vi "hadamard.vi"(1 "N":u16) -> (0 "Intensity Graph":dbl[][](graph))   [LabVIEW 2023]
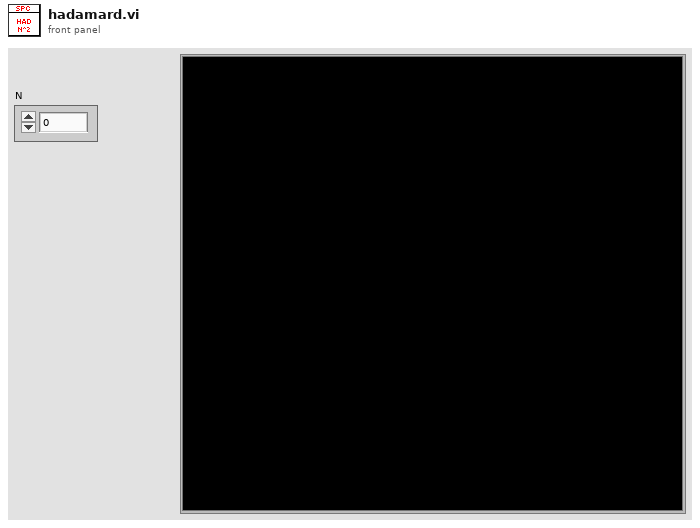
[diagram p1: front panel]
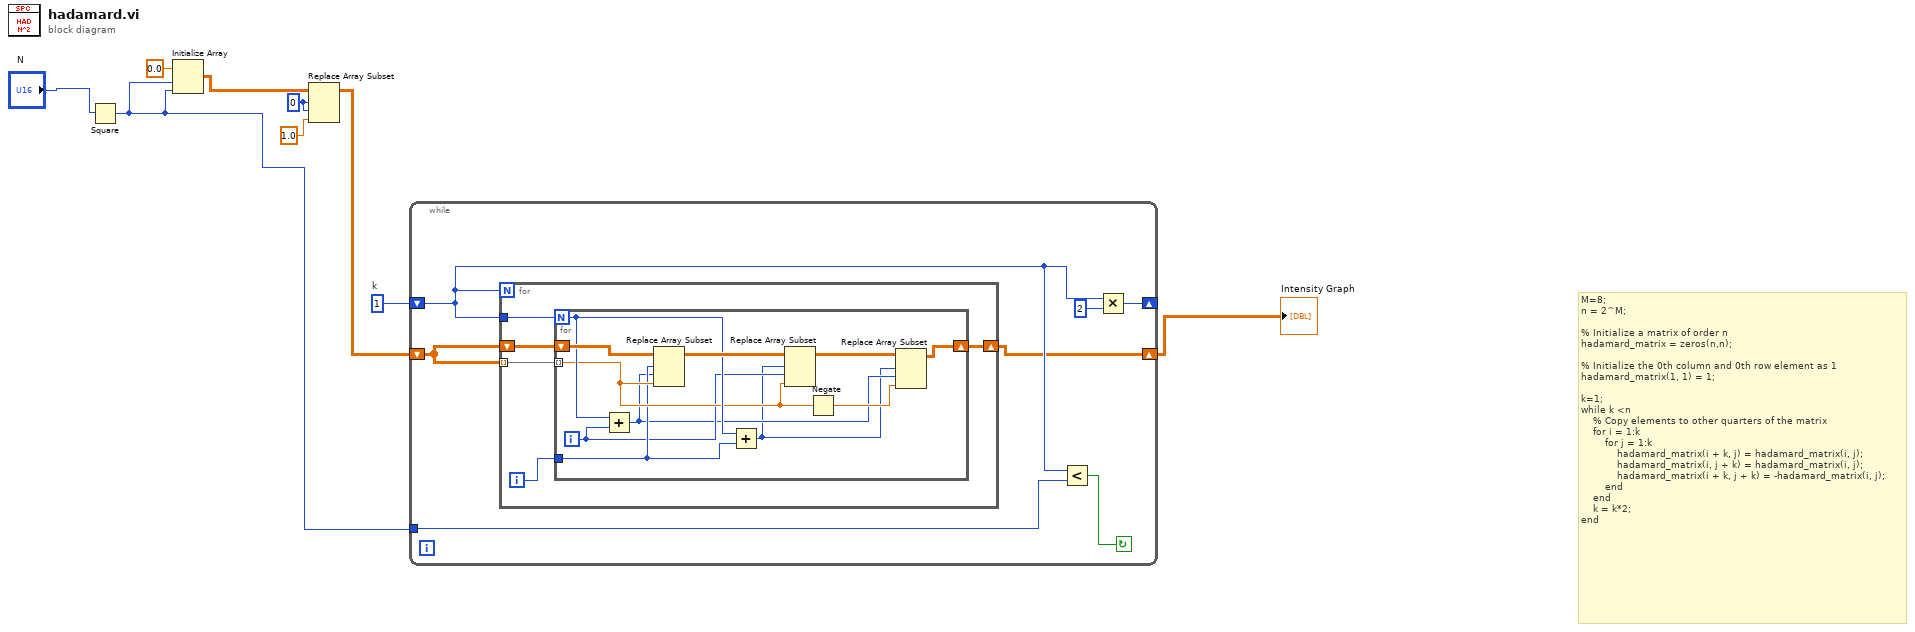
[diagram p0: block diagram]
diagram:
  w4 = 1  # k
  w6 = 0 ("index (row)")
  # "M=8;\nn = 2^M;\n\n% Initialize a matrix of order n\nhadamard_matrix = zeros(n,n);\n\n% Initialize the 0th column and 0th row element as 1\nhadamard_matrix(1, 1) = 1;\n\nk=1;\nwhile k <n\n    % Copy elements to other quarters of the matrix\n    for i = 1:k\n        for j = 1:k\n            hadamard_matrix(i + k, j) = hadamard_matrix(i, j);\n            hadamard_matrix(i, j + k) = hadamard_matrix(i, j);\n            hadamard_matrix(i + k, j + k) = -hadamard_matrix(i, j);\n        end\n    end\n    k = k*2;\nend"
  n1 = Square(x="N") -> (x^2=w2:u16)
  n2 = Initialize Array(0.0 ("element"), w2, w2) -> (w7:dbl[][])
  n3 = Replace Array Subset(array=w7, new element=1.0 ("new element/subarray"), index (row)=w6, index (col)=w6) -> (w3:dbl[][])
  n4 = while {
    shift-right: [w10] -> w1
    shift-left: w3 -> [w16]
    shift-right: [w11] -> _
    shift-left: w4 -> [w13]
    tunnel: w2 -> [w15]
    stop <- w14 continue-if-true
    n5 = for {
      N: w13 -> [_]
      tunnel: w13 -> [w21]
      tunnel: w16 -> [w19] mode=indexing
      shift-right: [w18] -> w10
      shift-left: w16 -> [w20]
      i -> [w17]
      n6 = for {
        N: w21 -> [w30]
        tunnel: w19 -> [w28] mode=indexing
        shift-right: [w26] -> w18
        shift-left: w20 -> [w32]
        tunnel: w17 -> [w25]
        i -> [w24]
        n7 = Add(x=w30, y=w24) -> (x+y=w23:i32)
        n8 = Replace Array Subset(array=w32, new element=w28, index (row)=w25, index (col)=w23) -> (w31:dbl[][])
        n9 = Add(x=w30, y=w25) -> (x+y=w22:i32)
        n10 = Replace Array Subset(array=w31, new element=w28, index (row)=w22, index (col)=w24) -> (w29:dbl[][])
        n11 = Negate(x=w28) -> (-x=w27:dbl)
        n12 = Replace Array Subset(array=w29, new element=w27, index (row)=w22, index (col)=w23) -> (w26:dbl[][])
      }
    }
    n13 = Less?(x=w13, y=w15) -> (x < y?=w14:bool)
    n14 = Multiply(x=w13, y=2) -> (x*y=w11:i32)
  }
  "Intensity Graph" <- w1
